vi "S2C_InstrClose.vi"(8 "Error In":errorcluster) -> (0 "Error Out":errorcluster)   [LabVIEW 2015]
doc: "Closes all instrument handles and references."
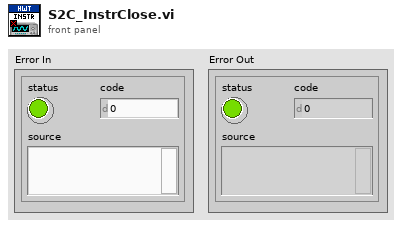
[diagram p1: front panel]
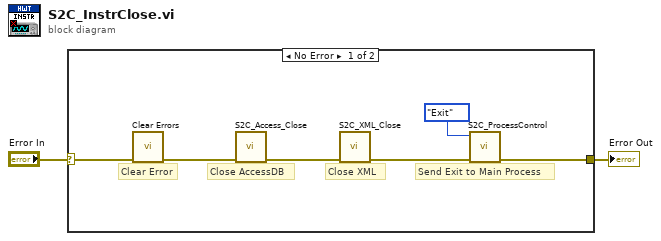
[diagram p0: block diagram]
diagram:
  n1 = case shown="No Error" "Error In" {
    selector: "Error In" -> [w6 w9]
    tunnel: [w8 w9] -> w2
    frame No Error {
      # "Close XML"
      # "Close AccessDB"
      # "Send Exit to Main Process"
      # "Clear Error"
      n2 = call <vilib>:"Clear Errors.vi"("error in (no error)"=w6) -> ("error out"=w5:errorcluster)  [unwired: 5 in, 1 out]
      n3 = call "S2C_Access_Close.vi"("Error In"=w5) -> ("Error Out"=w4:errorcluster)  [unwired: 10 in]
      n4 = call "S2C_XML_Close.vi"("Error In"=w4) -> ("Error Out"=w3:errorcluster)  [unwired: 10 in]
      n5 = call "S2C_ProcessControl.vi"("Error In"=w3, "Action"=enum16{"Launch", "Exit"}."Exit") -> ("Error Out"=w8:errorcluster)  [unwired: 9 in]
    }
    frame Error {
    }
  }
  "Error Out" <- w2
